vi "pumpcmd.vi"(7 "LabVIEW Web Service Request":refnum<class "Web Request.lvclass">) -> ()   [LabVIEW 2019]
uses:
  <vilib>/wsapi/Web Request.lvclass
  Controls/Test Action.ctl
panel:
  # "Use the Web Service Request input terminal to call the VIs on the Web Services palette. Do not remove it from the connector pane unless you don't need access to the palette."
  # "Each additional control wired to the connector pane will be available as an input in the URL. To include an indicator in terminal-mode output (the default setting), it must also be wired to the connector pane."
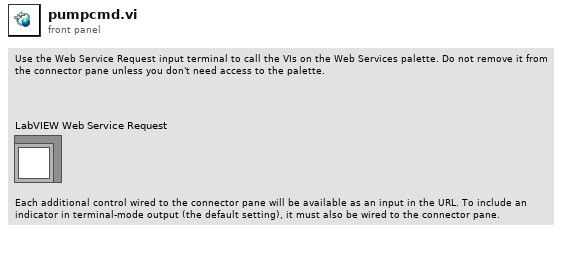
[diagram p1: front panel]
types:
  T1 = typedef "Test Action.ctl" = enum16{"Idle", "Start", "Stop", "Pump Cmd", "Pump 1 Enable", "Pump 2 Enable", "Pump 3 Enable", "Pump 4 Enable", "Pump 5 Enable", "Pump 6 Enable", "Timer 1 Reset", "Timer 2 Reset", "Timer 3 Reset", "Timer 4 Reset", "Timer 5 Reset", "Timer 6 Reset"}
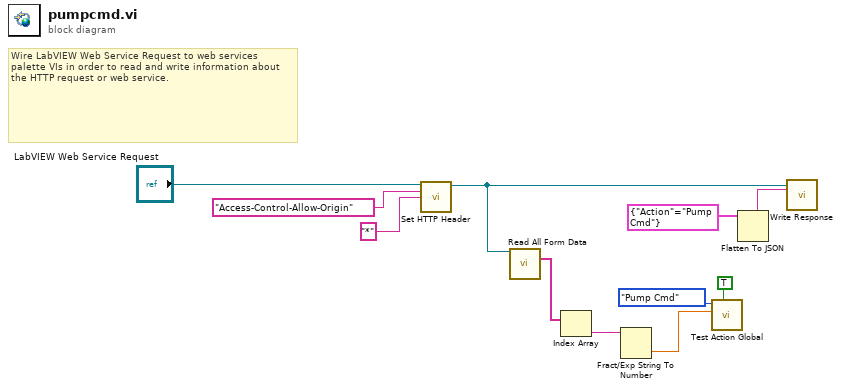
[diagram p0: block diagram]
diagram:
  # "Wire LabVIEW Web Service Request to web services palette VIs in order to read and write information about the HTTP request or web service."
  n1 = call <vilib>:"Set HTTP Header.vi"("LabVIEW Web Service Request"="LabVIEW Web Service Request", "header"="Access-Control-Allow-Origin" ("header value"), "header value"="*" ("header")) -> ("LabVIEW Web Service Request out"=w4:refnum<class "Web Request.lvclass">)  [unwired: 11 in, 1 out]
  n2 = call <vilib>:"Read All Form Data.vi"("LabVIEW Web Service Request"=w4) -> ("Key"=w3:string[])  [unwired: 10 in, 4 out]
  n3 = Index Array(array=w3) -> (element=w2:string)  [unwired: 1 in]
  n4 = Fract/Exp String To Number(string=w2) -> (number=w1:dbl)  [unwired: 3 in, 1 out]
  n5 = call "Test Action Global.vi"("Write (F)"=TRUE, "Data IN"=w1, "Test Action IN"=Test_Action."Pump Cmd") -> ()  [unwired: 7 in, 2 out]
  n6 = Flatten To JSON(anything=cluster{"Action":string} {"Action"="Pump Cmd"}) -> (JSON string=w8:string)  [unwired: 2 in, 1 out]
  n7 = call <vilib>:"Write Response.vi"("LabVIEW Web Service Request"=w4, "response string"=w8) -> ()  [unwired: 12 in, 2 out]
